vi "Set Decoration Label.vi"(4 "error in":errorcluster, 6 "Label":string, 7 "Decor Refnum":refnum<vi>) -> (0 "error out":errorcluster, 3 "dup Decor Refnum":refnum<vi>)   [LabVIEW 2020]
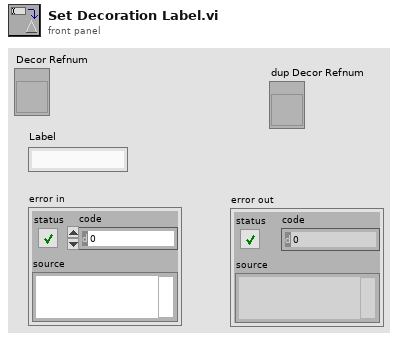
[diagram p1: front panel]
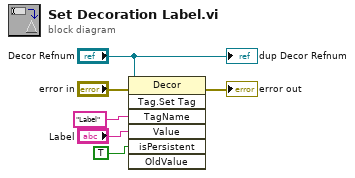
[diagram p0: block diagram]
diagram:
  n1 = invoke class="Decor" method="Tag.Set Tag"(reference="Decor Refnum", error in="error in", "TagName"="Label" ("Tag Name"), "Value"="Label", "isPersistent"=TRUE ("Is Persistent?")) -> (error out=→"error out":errorcluster)  [unwired: 2 in, 6 out]
  "dup Decor Refnum" <- "Decor Refnum"
